vi "MeasurmentVelocity.vi"() -> ()   [LabVIEW 2015]
uses:
  Control/AccelerationState.ctl
  <vilib>/DAQmx/write.llb/DAQmx Write (Analog 1D DBL NChan 1Samp).vi
  <vilib>/DAQmx/read.llb/DAQmx Read (Analog 1D DBL NChan 1Samp).vi
  <vilib>/DAQmx/create/channels.llb/DAQmx Create Channel (AO-Voltage-Basic).vi
  <vilib>/DAQmx/create/channels.llb/DAQmx Create Channel (AI-Voltage-Basic).vi
  <vilib>/DAQmx/miscellaneous.llb/DAQmx Fill In Error Info.vi
panel:
  out "Waveform Chart":u32(graph)
  out "String":string="0.0km/h"
  in  "DAQDevice":tag
  in  "Stop":bool
  in  "Ready":bool
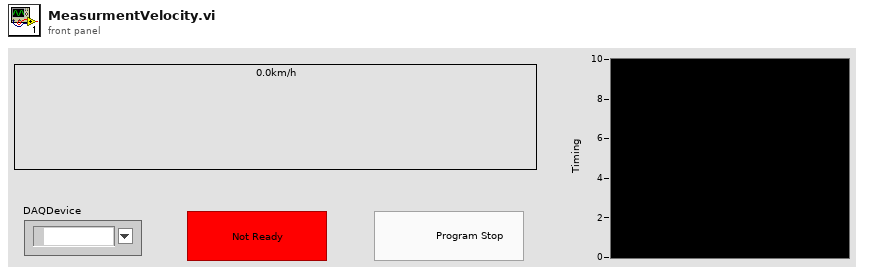
[diagram p1: front panel]
types:
  T1 = typedef "AccelerationState.ctl" = enum16{"Initial", "InputInfomation", "Ready", "Running", "FinshRunning", "LogRecord", "HardwareRelease", "RenewBestRecord", "ProgramStop"}
  T2 = cluster{"RefTime(ms)":i64, "Time(ms)":i64, "Distance(m)":dbl, "Velocity(km/h)":dbl, "Message":string, "State":T1}
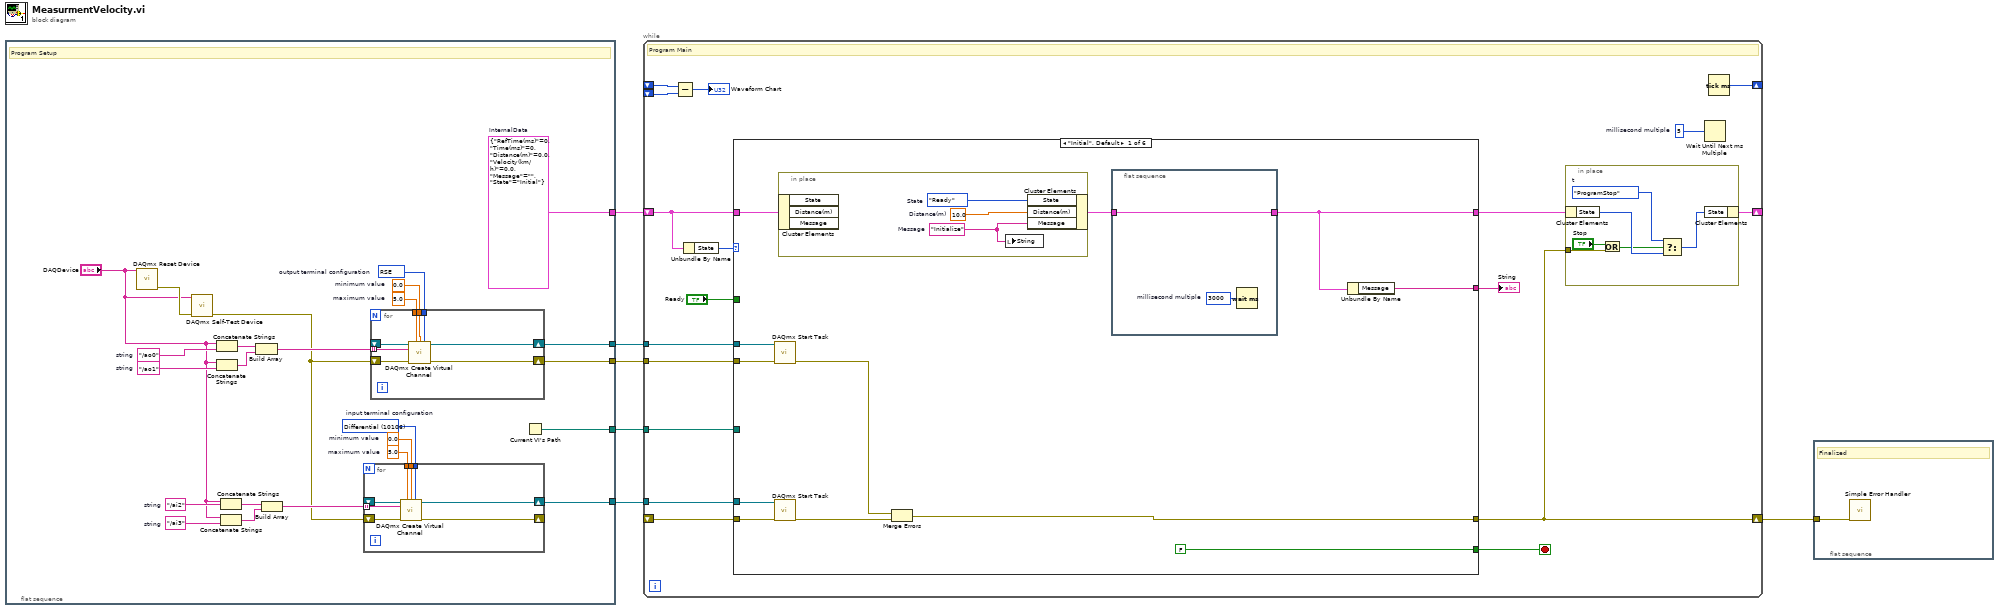
[diagram p0: block diagram]
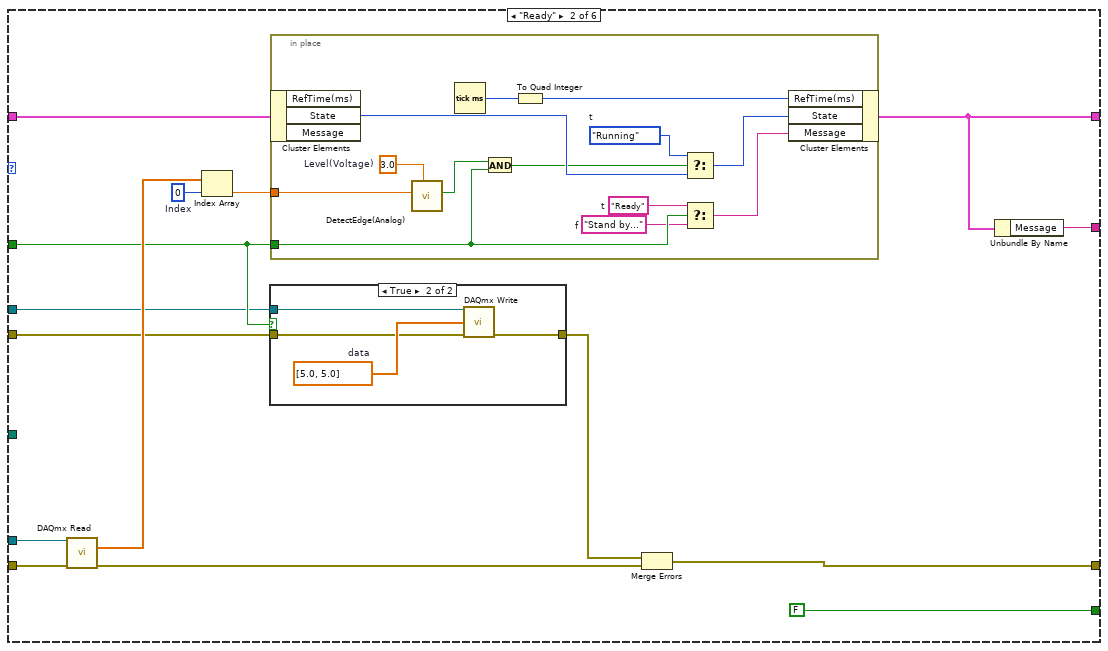
[diagram p2: hidden frame]
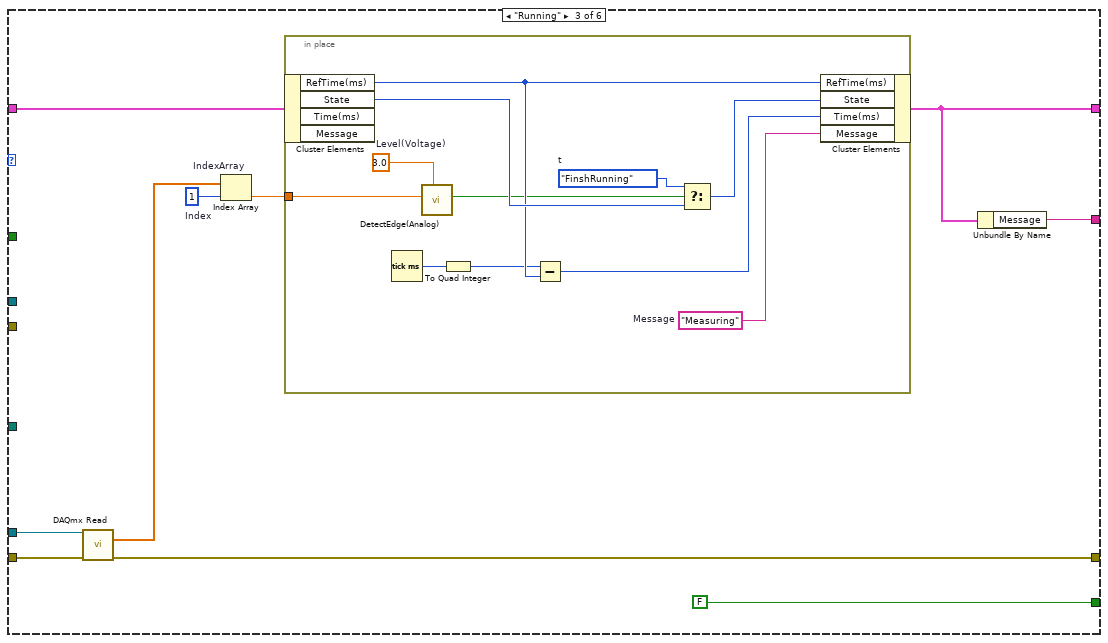
[diagram p4: hidden frame]
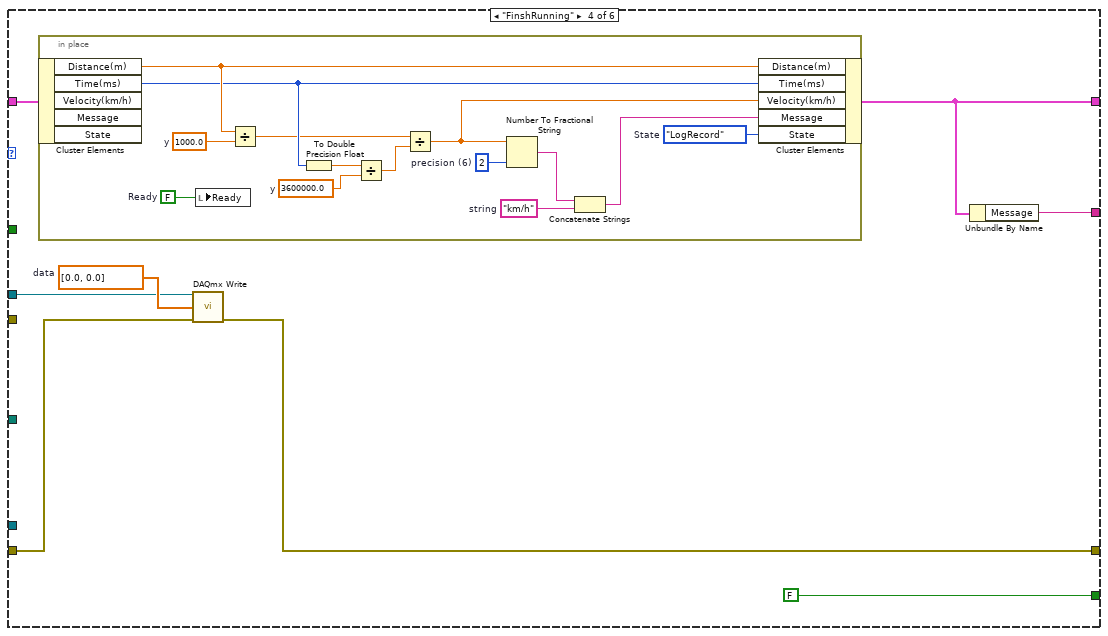
[diagram p5: hidden frame]
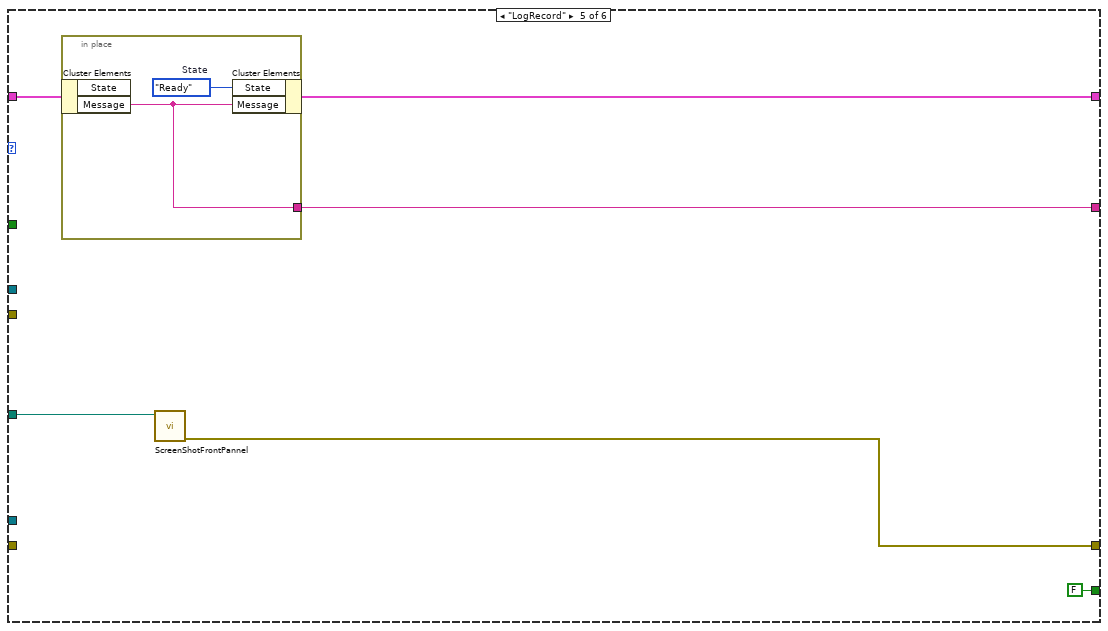
[diagram p6: hidden frame]
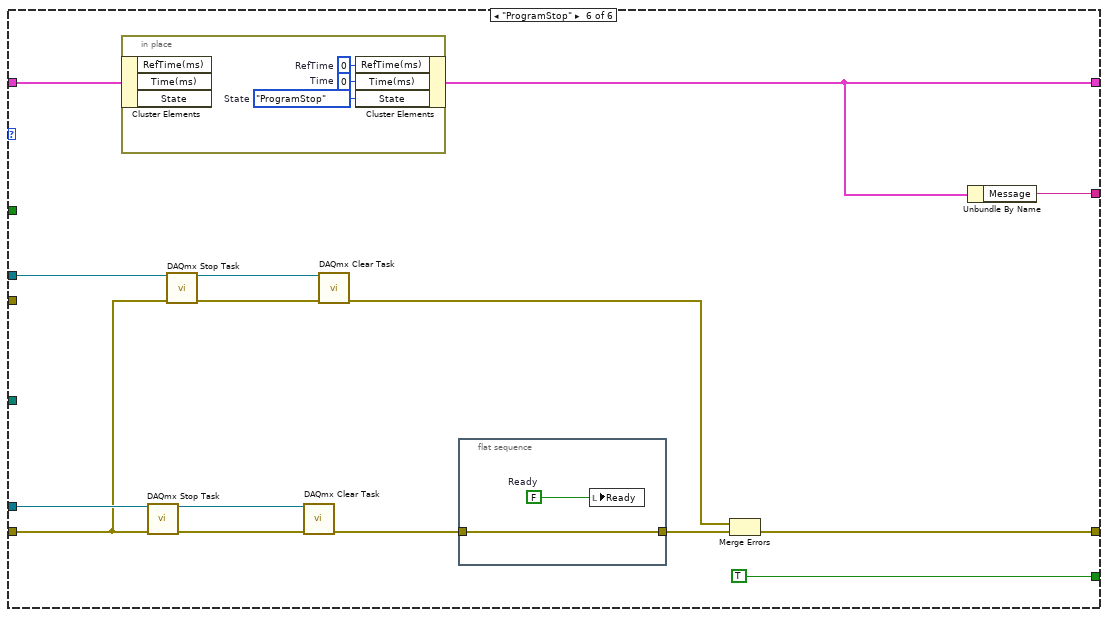
[diagram p7: hidden frame]
diagram:
  n1 = flat-sequence {
    tunnel: [w30] -> w5
    tunnel: [w28] -> w4
    tunnel: [w9] -> w3
    tunnel: [w8] -> w2
    tunnel: [w7] -> w1
    frame #0 {
      w9 = T2 {"RefTime(ms)"=0, "Time(ms)"=0, "Distance(m)"=0.0, "Velocity(km/h)"=0.0, "Message"="", "State"=enum."Initial"}  # InternalData
      w15 = "/ai3"  # string
      w16 = "/ai2"  # string
      w18 = "/ao1"  # string
      w20 = "/ao0"  # string
      w22 = 5.0  # maximum value
      w21 = 0.0  # minimum value
      w23 = 10106 items=["default"=-1, "RSE"=10083, "NRSE"=10078, "Differential"=10106, "Pseudodifferential"=12529]  # input terminal configuration
      w24 = 10083 items=["Default"=-1, "RSE"=10083, "Differential"=10106, "Pseudodifferential"=12529]  # output terminal configuration
      w25 = 0.0  # minimum value
      w26 = 5.0  # maximum value
      # "Program Setup"
      n2 = call <vilib>:"DAQmx Reset Device.vi"("device in"="DAQDevice") -> ("error out"=w12:errorcluster)  [unwired: 14 in]
      n3 = call <vilib>:"DAQmx Self-Test Device.vi"("device in"="DAQDevice", "error in"=w12) -> ("error out"=w10:errorcluster)  [unwired: 13 in]
      n4 = Concatenate Strings "Concatenate Strings"("DAQDevice", w20) -> (w19:string)
      n5 = Concatenate Strings "Concatenate Strings"("DAQDevice", w18) -> (w17:string)
      n6 = Concatenate Strings "Concatenate Strings"("DAQDevice", w16) -> (w14:string)
      n7 = Concatenate Strings "Concatenate Strings"("DAQDevice", w15) -> (w13:string)
      n8 = Build Array "Build Array"(w19, w17) -> (w27:string[])
      n9 = Build Array "Build Array"(w14, w13) -> (w29:string[])
      n10 = for {
        tunnel: w23 -> [w46]
        shift-right: [w45] -> _
        shift-left: w10 -> [w42]
        shift-right: [w44] -> w30
        shift-left: _ -> [w43]
        tunnel: w22 -> [w41]
        tunnel: w21 -> [w40]
        tunnel: w29 -> [w39] mode=indexing
        n11 = call-poly <vilib>:"DAQmx Create Virtual Channel.vi"("task in"=w43, "maximum value"=w41, "minimum value"=w40, "input terminal configuration"=w46, "physical channels"=w39, "error in"=w42) -> ("task out"=w44:refnum<k21>, "error out"=w45:errorcluster)  [unwired: 8 in]
      }
      n12 = for {
        shift-right: [w38] -> w28
        shift-left: _ -> [w35]
        shift-right: [w37] -> w8
        shift-left: w10 -> [w34]
        tunnel: w27 -> [w36] mode=indexing
        tunnel: w26 -> [w33]
        tunnel: w25 -> [w32]
        tunnel: w24 -> [w31]
        n13 = call-poly <vilib>:"DAQmx Create Virtual Channel.vi"("task in"=w35, "maximum value"=w33, "minimum value"=w32, "output terminal configuration"=w31, "physical channels"=w36, "error in"=w34) -> ("task out"=w38:refnum<k21>, "error out"=w37:errorcluster)  [unwired: 8 in]
      }
      n14 = Current VI's Path() -> (path=w7:path)
    }
  }
  n15 = while {
    tunnel: w5 -> [w64]
    shift-right: [w59] -> _
    shift-left: w3 -> [w61]
    shift-right: [w54] -> w6
    shift-left: _ -> [w63]
    tunnel: w4 -> [w56]
    tunnel: w2 -> [w53]
    shift-right: [w51] -> _
    shift-left: _ -> [w50]
    shift-left: _ -> [w49]
    tunnel: w1 -> [w47]
    stop <- w58 stop-if-true
    w55 = u32 5  # millisecond multiple
    # "Program Main"
    n16 = Subtract(x=w50, y=w49) -> (x-y=→"Waveform Chart":u32)
    n17 = Unbundle By Name(w61) -> ("State"=w62:T1)
    n18 = case shown="\"Initial\", Default" w62 {
      tunnel: w64 -> [w78 w102 w130 _ _ w184]
      tunnel: w63 -> [w77 w101 w129 w145 _ w175]
      tunnel: w61 -> [w82 w100 w126 w148 w166 w185]
      tunnel: [w72 w89 w122 w143 w165 w173] -> w60
      tunnel: [FALSE FALSE FALSE FALSE FALSE TRUE] -> w58
      tunnel: [w75 w91 w125 w144 w168 w180] -> w54
      tunnel: "Ready" -> [_ w94 _ _ _ _]
      tunnel: w56 -> [w80 w93 _ w146 _ w181]
      tunnel: w53 -> [w79 w92 _ _ _ _]
      tunnel: [w73 w88 w121 w142 w164 w172] -> w52
      tunnel: w47 -> [_ _ _ _ w169 _]
      frame "Initial", Default {
        n19 = call <vilib>:"DAQmx Start Task.vi"("task/channels in"=w80, "error in"=w79) -> ("error out"=w74:errorcluster)  [unwired: 12 in, 1 out]
        n20 = call <vilib>:"DAQmx Start Task.vi"("task/channels in"=w78, "error in"=w77) -> ("error out"=w76:errorcluster)  [unwired: 12 in, 1 out]
        n21 = in-place {
          w85 = "Initialize"  # Message
          w86 = 10.0  # Distance(m)
          w87 = AccelerationState."Ready"  # State
          n22 = in-place-cluster #1(w82) -> ()  [unwired: 3 out]
          n23 = local write "String"(w85) -> ()
          n24 = in-place-cluster #1("State"=w87, "Distance(m)"=w86, "Message"=w85) -> (w71:T2)
        }
        n25 = Merge Errors "Merge Errors"(w74, w76) -> (w75:errorcluster)
        n26 = flat-sequence {
          tunnel: [w84] -> w72
          tunnel: w71 -> [w84]
          frame #0 {
            w83 = u32 3000  # millisecond multiple
            n27 = Wait (ms)(milliseconds to wait=w83) -> ()  [unwired: 1 out]
          }
        }
        n28 = Unbundle By Name(w72) -> ("Message"=w73:string)
      }
      frame "Ready" {
        w98 = 0  # Index
        n29 = call-poly <vilib>:"DAQmx Read.vi"("task/channels in"=w102, "error in"=w101) -> ("data"=w97:dbl[], "error out"=w99:errorcluster)  [unwired: 11 in, 1 out]
        n30 = Index Array "Index Array"(array=w97, index=w98) -> (element=w96:dbl)
        n31 = case shown="True" w94 {
          tunnel: w93 -> [_ w107]
          tunnel: w92 -> [w103 w105]
          tunnel: [w103 w104] -> w90
          frame False {
          }
          frame True {
            w106 = dbl[] [5.0, 5.0]  # data
            n32 = call-poly <vilib>:"DAQmx Write.vi"("task/channels in"=w107, "data"=w106, "error in"=w105) -> ("error out"=w104:errorcluster)  [unwired: 10 in, 2 out]
          }
        }
        n33 = in-place {
          in-place-border: w96 -> [w117]
          in-place-border: w94 -> [w109]
          w108 = "Stand by..."  # f
          w110 = "Ready"  # t
          w115 = 3.0  # Level(Voltage)
          w119 = AccelerationState."Running"  # t
          n34 = in-place-cluster #2(w100) -> ("State"=w120:T1)  [unwired: 2 out]
          n35 = call "DetectEdge(Analog).vi"("Level(Voltage)"=w115, "Voltage"=w117) -> ("DetectedEdge"=w118:bool)  [unwired: 9 in]
          n36 = Tick Count (ms)() -> (millisecond timer value=w116:u32)
          n37 = And(x=w118, y=w109) -> (x .and. y?=w111:bool)
          n38 = To Quad Integer(1:w116) -> (0:w114:i64)
          n39 = Select(t=w119, s=w111, f=w120) -> (s? t:f=w113:T1)
          n40 = Select(t=w110, s=w109, f=w108) -> (s? t:f=w112:string)
          n41 = in-place-cluster #2("RefTime(ms)"=w114, "State"=w113, "Message"=w112) -> (w89:T2)
        }
        n42 = Merge Errors "Merge Errors"(w90, w99) -> (w91:errorcluster)
        n43 = Unbundle By Name(w89) -> ("Message"=w88:string)
      }
      frame "Running" {
        w124 = 1  # Index
        n44 = call-poly <vilib>:"DAQmx Read.vi"("task/channels in"=w130, "error in"=w129) -> ("data"=w128:dbl[], "error out"=w125:errorcluster)  [unwired: 11 in, 1 out]
        n45 = Index Array "IndexArray"(array=w128, index=w124) -> (element=w123:dbl)
        n46 = in-place {
          in-place-border: w123 -> [w136]
          w131 = "Measuring"  # Message
          w134 = 3.0  # Level(Voltage)
          w140 = AccelerationState."FinshRunning"  # t
          n47 = in-place-cluster #3(w126) -> ("RefTime(ms)"=w138:i64, "State"=w141:T1)  [unwired: 2 out]
          n48 = Tick Count (ms)() -> (millisecond timer value=w139:u32)
          n49 = call "DetectEdge(Analog).vi"("Level(Voltage)"=w134, "Voltage"=w136) -> ("DetectedEdge"=w135:bool)  [unwired: 9 in]
          n50 = To Quad Integer(1:w139) -> (0:w133:i64)
          n51 = Subtract(x=w133, y=w138) -> (x-y=w132:i64)
          n52 = Select(t=w140, s=w135, f=w141) -> (s? t:f=w137:T1)
          n53 = in-place-cluster #3("RefTime(ms)"=w138, "State"=w137, "Time(ms)"=w132, "Message"=w131) -> (w122:T2)
        }
        n54 = Unbundle By Name(w122) -> ("Message"=w121:string)
      }
      frame "FinshRunning" {
        w147 = dbl[] [0.0, 0.0]  # data
        n55 = in-place {
          w154 = "km/h"  # string
          w152 = i16 2  # precision (6)
          w158 = 3600000.0  # y
          w159 = 1000.0  # y
          w162 = FALSE  # Ready
          w163 = AccelerationState."LogRecord"  # State
          n56 = in-place-cluster #4(w148) -> ("Distance(m)"=w161:dbl, "Time(ms)"=w160:i64)  [unwired: 3 out]
          n57 = local write "Ready"(w162) -> ()
          n58 = Divide(x=w161, y=w159) -> (x/y=w157:dbl)
          n59 = To Double Precision Float(number=w160) -> (double precision float=w155:dbl)
          n60 = Divide(x=w155, y=w158) -> (x/y=w156:dbl)
          n61 = Divide(x=w157, y=w156) -> (x/y=w150:dbl)
          n62 = Number To Fractional String(number=w150, precision (6)=w152) -> (F-format string=w153:string)  [unwired: 2 in]
          n63 = Concatenate Strings "Concatenate Strings"(w153, w154) -> (w151:string)
          n64 = in-place-cluster #4("Distance(m)"=w161, "Time(ms)"=w160, "Velocity(km/h)"=w150, "Message"=w151, "State"=w163) -> (w143:T2)
        }
        n65 = call-poly <vilib>:"DAQmx Write.vi"("task/channels in"=w146, "data"=w147, "error in"=w145) -> ("error out"=w144:errorcluster)  [unwired: 10 in, 2 out]
        n66 = Unbundle By Name(w143) -> ("Message"=w142:string)
      }
      frame "LogRecord" {
        n67 = in-place {
          in-place-border: [w170] -> w164
          w171 = AccelerationState."Ready"  # State
          n68 = in-place-cluster #5(w166) -> ("Message"=w170:string)  [unwired: 1 out]
          n69 = in-place-cluster #5("State"=w171, "Message"=w170) -> (w165:T2)
        }
        n70 = call "ScreenShotFrontPannel.vi"("vi path"=w169) -> ("error out"=w168:errorcluster)  [unwired: 10 in]
      }
      frame "ProgramStop" {
        n71 = in-place {
          w189 = AccelerationState."ProgramStop"  # State
          w190 = i64 0  # RefTime
          w191 = i64 0  # Time
          n72 = in-place-cluster #6(w185) -> ()  [unwired: 3 out]
          n73 = in-place-cluster #6("RefTime(ms)"=w190, "Time(ms)"=w191, "State"=w189) -> (w173:T2)
        }
        n74 = call <vilib>:"DAQmx Stop Task.vi"("task/channels in"=w184, "error in"=w175) -> ("task out"=w177:refnum<k21>, "error out"=w176:errorcluster)  [unwired: 12 in]
        n75 = call <vilib>:"DAQmx Stop Task.vi"("task/channels in"=w181, "error in"=w175) -> ("task out"=w178:refnum<k21>, "error out"=w174:errorcluster)  [unwired: 12 in]
        n76 = call <vilib>:"DAQmx Clear Task.vi"("task in"=w177, "error in"=w176) -> ("error out"=w183:errorcluster)  [unwired: 13 in]
        n77 = call <vilib>:"DAQmx Clear Task.vi"("task in"=w178, "error in"=w174) -> ("error out"=w179:errorcluster)  [unwired: 13 in]
        n78 = flat-sequence {
          tunnel: w183 -> [w188]
          tunnel: [w188] -> w182
          frame #0 {
            w187 = FALSE  # Ready
            n79 = local write "Ready"(w187) -> ()
          }
        }
        n80 = Merge Errors "Merge Errors"(w179, w182) -> (w180:errorcluster)
        n81 = Unbundle By Name(w173) -> ("Message"=w172:string)
      }
    }
    "String" <- w52
    n82 = in-place {
      in-place-border: w54 -> [w65]
      w67 = AccelerationState."ProgramStop"  # t
      n83 = in-place-cluster #7(w60) -> ("State"=w69:T1)
      n84 = Or(x="Stop", y=w65) -> (x .or. y?=w66:bool)
      n85 = Select(t=w67, s=w66, f=w69) -> (s? t:f=w68:T1)
      n86 = in-place-cluster #7("State"=w68) -> (w59:T2)
    }
    n87 = Wait Until Next ms Multiple(millisecond multiple=w55) -> ()  [unwired: 1 out]
    n88 = Tick Count (ms)() -> (millisecond timer value=w51:u32)
  }
  n89 = flat-sequence {
    tunnel: w6 -> [w192]
    frame #0 {
      # "Finalized"
      n90 = call <vilib>:"Simple Error Handler.vi"("error in (no error)"=w192) -> ()  [unwired: 4 in, 5 out]
    }
  }
